vi "Engine-AnalogInputs-Host.vi"() -> ()   [LabVIEW 2016]
uses:
  <vilib>/addons/Software Calibration Management/XControls/TBL1D.xctl
panel:
  in  "_AIx_ExtPU":sgl caption="External Pullup [W]" format="%#_4p"
  in  "_Invisible":enum32{"Hidden Items"}(tab)
  in  "Unit":string[](array[string])
  in  "Name":string[](array[string])
  out "AI":sgl[](array[numeric])
  in  "SimE":bool[](array[boolean])
  in  "Sim":sgl[](array[numeric])
  in  "FiltE":bool[](array[boolean])
  in  "FiltCutoff":sgl[](array[numeric])
  out "AI_Raw":sgl[](array[numeric])
  in  "ExtPU":sgl[](array[numeric])
  in  "_Table Tab Ctrl":T1(tab)
  in  "AI01_Tbl":cluster{"X":sgl[], "Y":sgl[]}(xcontrol) caption="[V|bar]"
  in  "AI02_Tbl":cluster{"X":sgl[], "Y":sgl[]}(xcontrol) caption="[V|bar]"
  in  "AI03_Tbl":cluster{"X":sgl[], "Y":sgl[]}(xcontrol) caption="[V|bar]"
  in  "AI04_Tbl":cluster{"X":sgl[], "Y":sgl[]}(xcontrol) caption="[V|bar]"
  in  "AI05_Tbl":cluster{"X":sgl[], "Y":sgl[]}(xcontrol) caption="[V|bar]"
  in  "AI06_Tbl":cluster{"X":sgl[], "Y":sgl[]}(xcontrol) caption="[V|bar]"
  in  "AI07_Tbl":cluster{"X":sgl[], "Y":sgl[]}(xcontrol) caption="[V|bar]"
  in  "AI08_Tbl":cluster{"X":sgl[], "Y":sgl[]}(xcontrol) caption="[V|bar]"
  in  "AI09_Tbl":cluster{"X":sgl[], "Y":sgl[]}(xcontrol) caption="[V|bar]"
  in  "AI10_Tbl":cluster{"X":sgl[], "Y":sgl[]}(xcontrol) caption="[V|bar]"
  in  "AI11_Tbl":cluster{"X":sgl[], "Y":sgl[]}(xcontrol) caption="[V|bar]"
  in  "AI12_Tbl":cluster{"X":sgl[], "Y":sgl[]}(xcontrol) caption="[V|bar]"
  in  "_AIx_FiltCutoff":sgl caption="Filter Cutoff [Hz]" format="%#_4p"
  in  "_AIx_FiltE":bool
  in  "_AIx_Sim":sgl caption="AIx_Sim"
  in  "_AIx_SimE":bool
  in  "_AIx_Name":string caption="AIx_Name"
  in  "_AIx_Unit":string caption="AIx_Unit"
  in  "_Analog Input Channel":i32(listbox) caption="Analog Inputs"
  # "W"
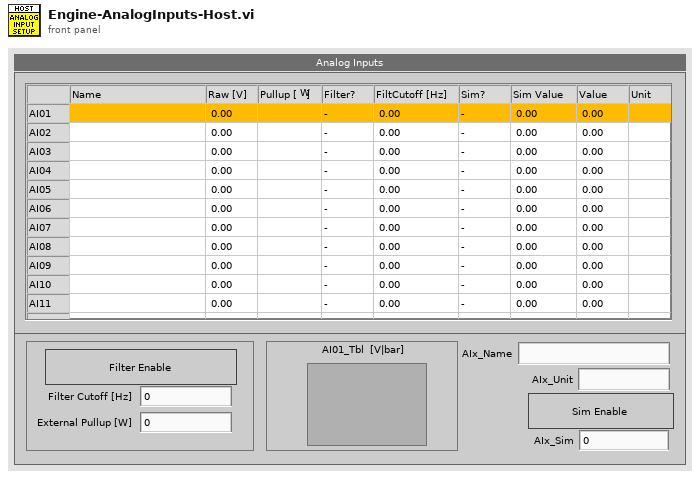
[diagram p1: front panel]
types:
  T1 = enum32{"AI01", "AI02", "AI03", "AI04", "AI05", "AI06", "AI07", "AI08", "AI09", "AI10", "AI11", "AI12"}
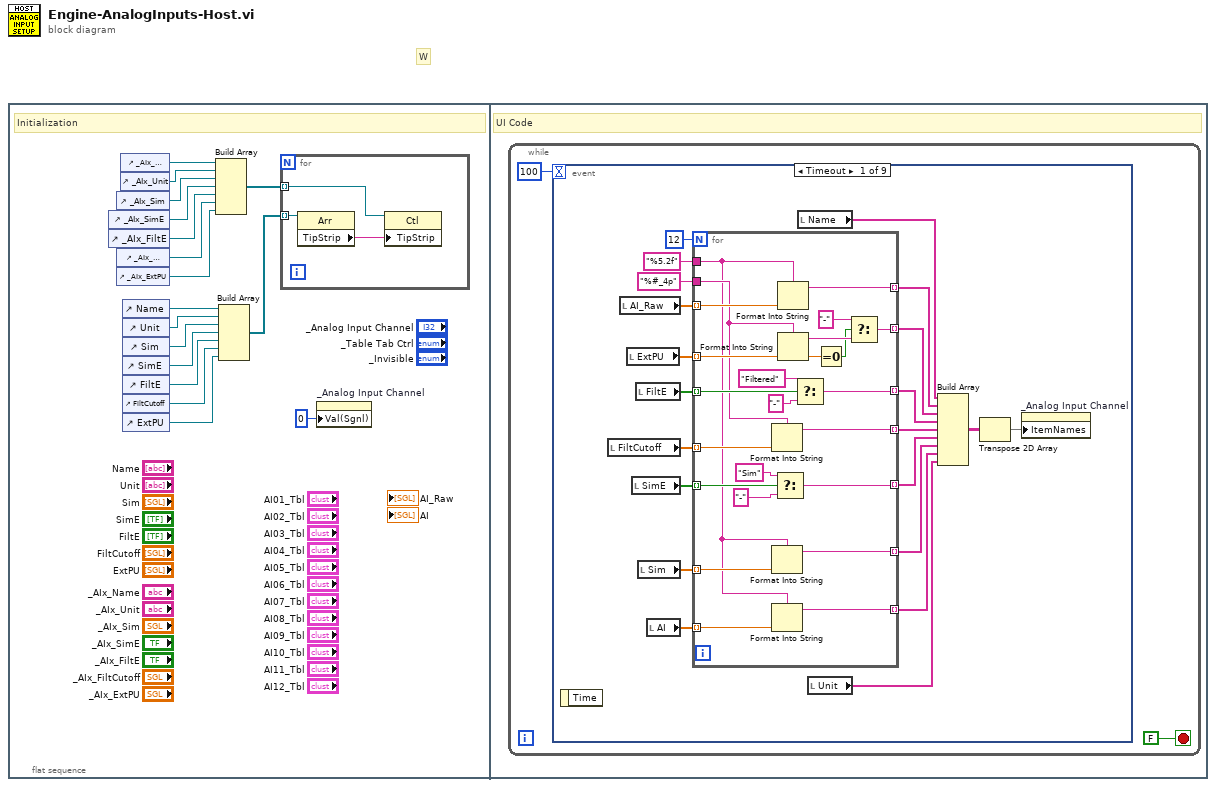
[diagram p0: block diagram]
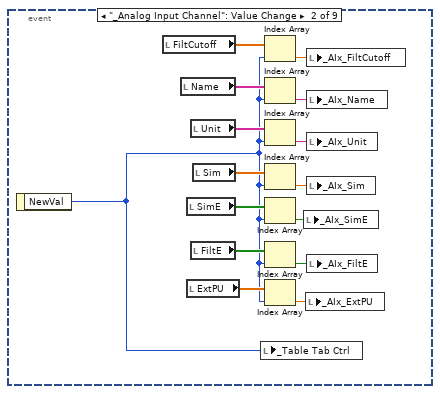
[diagram p2: hidden frame]
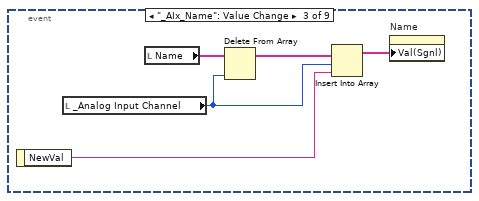
[diagram p3: hidden frame]
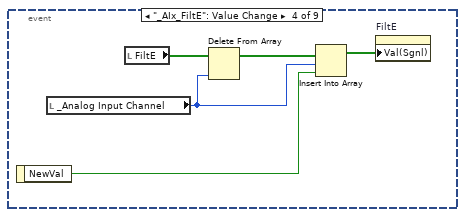
[diagram p4: hidden frame]
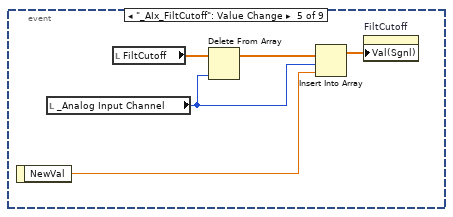
[diagram p5: hidden frame]
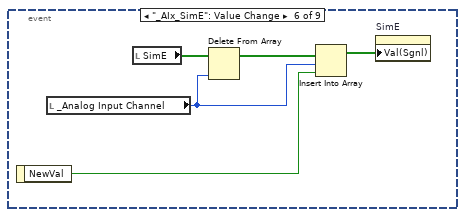
[diagram p6: hidden frame]
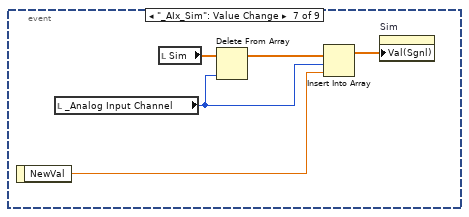
[diagram p7: hidden frame]
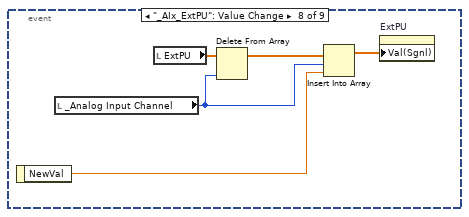
[diagram p8: hidden frame]
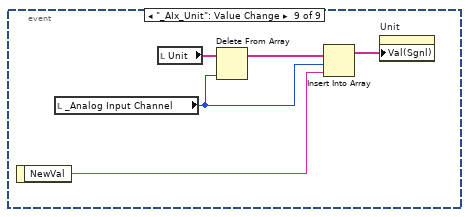
[diagram p9: hidden frame]
diagram:
  # "W"
  n1 = flat-sequence {
    frame #0 {
      # "Initialization"
      n2 = control-ref of="_AIx_SimE"() -> (w5:refnum<vi>)
      n3 = control-ref of="_AIx_FiltE"() -> (w4:refnum<vi>)
      n4 = control-ref of="_AIx_Sim"() -> (w6:refnum<vi>)
      n5 = control-ref of="_AIx_FiltCutoff"() -> (w3:refnum<vi>)
      n6 = control-ref of="_AIx_ExtPU"() -> (w2:refnum<vi>)
      n7 = control-ref of="_AIx_Name"() -> (w8:refnum<vi>)
      n8 = control-ref of="_AIx_Unit"() -> (w7:refnum<vi>)
      n9 = control-ref of="Name"() -> (w16:refnum<vi>)
      n10 = control-ref of="Unit"() -> (w15:refnum<vi>)
      n11 = control-ref of="Sim"() -> (w14:refnum<vi>)
      n12 = control-ref of="SimE"() -> (w13:refnum<vi>)
      n13 = control-ref of="FiltE"() -> (w12:refnum<vi>)
      n14 = control-ref of="FiltCutoff"() -> (w11:refnum<vi>)
      n15 = control-ref of="ExtPU"() -> (w10:refnum<vi>)
      n16 = Build Array(w8, w7, w6, w5, w4, w3, w2) -> (w1:refnum<vi>[])
      n17 = Build Array(w16, w15, w14, w13, w12, w11, w10) -> (w9:refnum<vi>[])
      n18 = for {
        tunnel: w9 -> [w20] mode=indexing
        tunnel: w1 -> [w18] mode=indexing
        n19 = property class="Arr"(reference=w20) -> ("TipStrip"=w19:string)  [unwired: 1 in, 2 out]
        n20 = property class="Ctl"(reference=w18, "TipStrip"=w19) -> ()  [unwired: 1 in, 2 out]
      }
      n21 = property on="_Analog Input Channel" class="MCListbox (strict)"("Val(Sgnl)"=0 ("Value (Signaling)")) -> ()  [unwired: 2 in, 2 out]
    }
    frame #1 {
      # "UI Code"
      n22 = while {
        stop <- FALSE stop-if-true
        n23 = event shown="[0] Timeout" {
          selector: _ -> [_ _ _ _ _ _ _ _ _]
          dyn-events: _ -> [_ _ _ _ _ _ _ _ _]
          timeout: 100 -> [_ _ _ _ _ _ _ _ _]
          event Timeout {
            n24 = event-data() -> ()  [unwired: 1 in, 1 out]
            n25 = local read "FiltCutoff"() -> (w35:sgl[])
            n26 = local read "AI_Raw"() -> (w37:sgl[])
            n27 = local read "ExtPU"() -> (w25:sgl[])
            n28 = local read "SimE"() -> (w34:bool[])
            n29 = local read "FiltE"() -> (w36:bool[])
            n30 = local read "Sim"() -> (w33:sgl[])
            n31 = local read "AI"() -> (w42:sgl[])
            n32 = for {
              N: 12 -> [_]
              tunnel: w42 -> [w65] mode=indexing
              tunnel: [w66] -> w41 mode=indexing
              tunnel: w37 -> [w57] mode=indexing
              tunnel: w36 -> [w63] mode=indexing
              tunnel: w35 -> [w62] mode=indexing
              tunnel: w34 -> [w59] mode=indexing
              tunnel: w33 -> [w58] mode=indexing
              tunnel: [w56] -> w28 mode=indexing
              tunnel: [w55] -> w29 mode=indexing
              tunnel: [w54] -> w30 mode=indexing
              tunnel: [w53] -> w31 mode=indexing
              tunnel: [w52] -> w32 mode=indexing
              tunnel: [w49] -> w26 mode=indexing
              tunnel: w25 -> [w46] mode=indexing
              tunnel: "%#_4p" ("format string") -> [w45]
              tunnel: "%5.2f" ("format string") -> [w44]
              n33 = Format Into String(format string=w45, w62) -> (resulting string=w54:string)  [unwired: 2 in, 1 out]
              n34 = Format Into String(format string=w44, w58) -> (resulting string=w56:string)  [unwired: 2 in, 1 out]
              n35 = Format Into String(format string=w44, w65) -> (resulting string=w66:string)  [unwired: 2 in, 1 out]
              n36 = Select(t="Sim" ("format string"), s=w59, f="-" ("format string")) -> (s? t:f=w55:string)
              n37 = Format Into String(format string=w44, w57) -> (resulting string=w52:string)  [unwired: 2 in, 1 out]
              n38 = Format Into String(format string=w45, w46) -> (resulting string=w50:string)  [unwired: 2 in, 1 out]
              n39 = Select(t="Filtered" ("format string"), s=w63, f="-" ("format string")) -> (s? t:f=w53:string)
              n40 = Equal To 0?(x=w46) -> (x = 0?=w47:bool)
              n41 = Select(t="-", s=w47, f=w50) -> (s? t:f=w49:string)
            }
            n42 = local read "Name"() -> (w38:string[])
            n43 = local read "Unit"() -> (w43:string[])
            n44 = Build Array(w38, w32, w26, w31, w30, w29, w28, w41, w43) -> (w40:string[][])
            n45 = Transpose 2D Array(2D array=w40) -> (transposed array=w39:string[][])
            n46 = property on="_Analog Input Channel" class="MCListbox (strict)"("ItemNames"=w39) -> ()  [unwired: 2 in, 2 out]
          }
          event "_Analog Input Channel": Value Change {
            n47 = event-data() -> ("NewVal"=w67:i32)  [unwired: 1 in]
            n48 = local read "FiltCutoff"() -> (w75:sgl[])
            n49 = local read "Name"() -> (w74:string[])
            n50 = local read "SimE"() -> (w71:bool[])
            n51 = local read "ExtPU"() -> (w68:sgl[])
            n52 = local read "Unit"() -> (w73:string[])
            n53 = local read "FiltE"() -> (w70:bool[])
            n54 = local read "Sim"() -> (w72:sgl[])
            n55 = local write "_Table Tab Ctrl"(w67) -> ()
            n56 = Index Array(array=w75, index=w67) -> (element=w78:sgl)
            n57 = Index Array(array=w74, index=w67) -> (element=w76:string)
            n58 = Index Array(array=w73, index=w67) -> (element=w81:string)
            n59 = Index Array(array=w72, index=w67) -> (element=w80:sgl)
            n60 = Index Array(array=w71, index=w67) -> (element=w79:bool)
            n61 = Index Array(array=w70, index=w67) -> (element=w77:bool)
            n62 = Index Array(array=w68, index=w67) -> (element=w69:sgl)
            n63 = local write "_AIx_SimE"(w79) -> ()
            n64 = local write "_AIx_ExtPU"(w69) -> ()
            n65 = local write "_AIx_FiltCutoff"(w78) -> ()
            n66 = local write "_AIx_Name"(w76) -> ()
            n67 = local write "_AIx_Unit"(w81) -> ()
            n68 = local write "_AIx_Sim"(w80) -> ()
            n69 = local write "_AIx_FiltE"(w77) -> ()
          }
          event "_AIx_Name": Value Change {
            n70 = event-data() -> ("NewVal"=w84:string)  [unwired: 1 in]
            n71 = local read "_Analog Input Channel"() -> (w85:i32)
            n72 = local read "Name"() -> (w83:string[])
            n73 = Delete From Array(array=w83, index=w85) -> (array with subset deleted=w86:string[])  [unwired: 1 in, 1 out]
            n74 = Insert Into Array(array=w86, index=w85, new element=w84) -> (w82:string[])
            n75 = property on="Name" class="Arr (strict)"("Val(Sgnl)"=w82) -> ()  [unwired: 2 in, 2 out]
          }
          event "_AIx_FiltE": Value Change {
            n76 = event-data() -> ("NewVal"=w89:bool)  [unwired: 1 in]
            n77 = local read "_Analog Input Channel"() -> (w90:i32)
            n78 = local read "FiltE"() -> (w88:bool[])
            n79 = Delete From Array(array=w88, index=w90) -> (array with subset deleted=w91:bool[])  [unwired: 1 in, 1 out]
            n80 = Insert Into Array(array=w91, index=w90, new element=w89) -> (w87:bool[])
            n81 = property on="FiltE" class="Arr (strict)"("Val(Sgnl)"=w87) -> ()  [unwired: 2 in, 2 out]
          }
          event "_AIx_FiltCutoff": Value Change {
            n82 = event-data() -> ("NewVal"=w94:sgl)  [unwired: 1 in]
            n83 = local read "_Analog Input Channel"() -> (w95:i32)
            n84 = local read "FiltCutoff"() -> (w93:sgl[])
            n85 = Delete From Array(array=w93, index=w95) -> (array with subset deleted=w96:sgl[])  [unwired: 1 in, 1 out]
            n86 = Insert Into Array(array=w96, index=w95, new element=w94) -> (w92:sgl[])
            n87 = property on="FiltCutoff" class="Arr (strict)"("Val(Sgnl)"=w92) -> ()  [unwired: 2 in, 2 out]
          }
          event "_AIx_SimE": Value Change {
            n88 = event-data() -> ("NewVal"=w99:bool)  [unwired: 1 in]
            n89 = local read "_Analog Input Channel"() -> (w100:i32)
            n90 = local read "SimE"() -> (w98:bool[])
            n91 = Delete From Array(array=w98, index=w100) -> (array with subset deleted=w101:bool[])  [unwired: 1 in, 1 out]
            n92 = Insert Into Array(array=w101, index=w100, new element=w99) -> (w97:bool[])
            n93 = property on="SimE" class="Arr (strict)"("Val(Sgnl)"=w97) -> ()  [unwired: 2 in, 2 out]
          }
          event "_AIx_Sim": Value Change {
            n94 = event-data() -> ("NewVal"=w104:sgl)  [unwired: 1 in]
            n95 = local read "_Analog Input Channel"() -> (w105:i32)
            n96 = local read "Sim"() -> (w103:sgl[])
            n97 = Delete From Array(array=w103, index=w105) -> (array with subset deleted=w106:sgl[])  [unwired: 1 in, 1 out]
            n98 = Insert Into Array(array=w106, index=w105, new element=w104) -> (w102:sgl[])
            n99 = property on="Sim" class="Arr (strict)"("Val(Sgnl)"=w102) -> ()  [unwired: 2 in, 2 out]
          }
          event "_AIx_ExtPU": Value Change {
            n100 = event-data() -> ("NewVal"=w109:sgl)  [unwired: 1 in]
            n101 = local read "_Analog Input Channel"() -> (w110:i32)
            n102 = local read "ExtPU"() -> (w108:sgl[])
            n103 = Delete From Array(array=w108, index=w110) -> (array with subset deleted=w111:sgl[])  [unwired: 1 in, 1 out]
            n104 = Insert Into Array(array=w111, index=w110, new element=w109) -> (w107:sgl[])
            n105 = property on="ExtPU" class="Arr (strict)"("Val(Sgnl)"=w107) -> ()  [unwired: 2 in, 2 out]
          }
          event "_AIx_Unit": Value Change {
            n106 = event-data() -> ("NewVal"=w114:string)  [unwired: 1 in]
            n107 = local read "_Analog Input Channel"() -> (w115:i32)
            n108 = local read "Unit"() -> (w113:string[])
            n109 = Delete From Array(array=w113, index=w115) -> (array with subset deleted=w116:string[])  [unwired: 1 in, 1 out]
            n110 = Insert Into Array(array=w116, index=w115, new element=w114) -> (w112:string[])
            n111 = property on="Unit" class="Arr (strict)"("Val(Sgnl)"=w112) -> ()  [unwired: 2 in, 2 out]
          }
        }
      }
    }
  }
